vi "Load Layout.vi"(4 "PlotPane":refnum<vi>, 5 "MultiPlotPanel in":refnum<class "MultiPlotPanel.lvclass">, 6 "Subpanel Refs (ALL)":refnum<vi>[](array[refnum]), 7 "RocketPlotPanel Type":refnum<class "RocketPlotPanel.lvclass">, 8 "error in (no error)":errorcluster, 10 "file extension":string, 11 "Loop data in":T1 {"PanelMap"."Data"."Plot Bounds (%)"."Bottom (%)" format="%.2f"; "PanelMap"."Data"."Plot Bounds (%)"."Top (%)" format="%.2f"; "PanelMap"."Data"."Plot Bounds (%)"."Right (%)" format="%.2f"; "PanelMap"."Data"."Plot Bounds (%)"."Left (%)" format="%.2f"}) -> (0 "error out":errorcluster, 1 "Valid load?":bool, 2 "Filename":string, 3 "Loop data out":T1 {"PanelMap"."Data"."Plot Bounds (%)"."Bottom (%)" format="%.2f"; "PanelMap"."Data"."Plot Bounds (%)"."Top (%)" format="%.2f"; "PanelMap"."Data"."Plot Bounds (%)"."Right (%)" format="%.2f"; "PanelMap"."Data"."Plot Bounds (%)"."Left (%)" format="%.2f"})   [LabVIEW 2021, in "MultiStokePlot.lvlib" / "MultiPlotPanel.lvclass"]
uses:
  Classes/MultiPlotPanel/MultiPlotPanel.lvclass
  Loop Data.ctl
  <vilib>/IlluminatedG/IG OOPanel/OOPanel/Manager/Manager.lvclass
  Panel Map.ctl
  Panel Map Data.ctl
  <userlib>/bjustice/RocketPlot/Classes/RocketPlotPanel/RocketPlotPanel.lvclass
  Window Position.ctl
  <vilib>/IlluminatedG/IG OOPanel/OOPanel/Panel/Panel Events.ctl
  <vilib>/IlluminatedG/IG OOPanel/OOPanel/Panel/Visbility Event Data.ctl
  <vilib>/IlluminatedG/IG OOPanel/OOPanel/Visibility State.ctl
  <vilib>/IlluminatedG/IG OOPanel/OOPanel/Close Reason.ctl
  Classes/MultiPlotPanel/MultiPlotPanel.lvclass/MultiPlotPanel.ctl
  Window Position and plot number.ctl
  <userlib>/bjustice/RocketPlot/Classes/RocketPlotPanel/RocketPlotPanel.lvclass/RocketPlotPanel.ctl
  <userlib>/bjustice/RocketPlot/Classes/RocketPlotPanel/Read RocketPlotHandle.vi
  <userlib>/bjustice/RocketPlot/Classes/RocketPlotHandle/RocketPlotHandle.lvclass
  <vilib>/IlluminatedG/IG OOPanel/OOPanel/OOPanel.lvlib
  <vilib>/IlluminatedG/IG OOPanel/OOPanel/Panel/Panel.lvclass
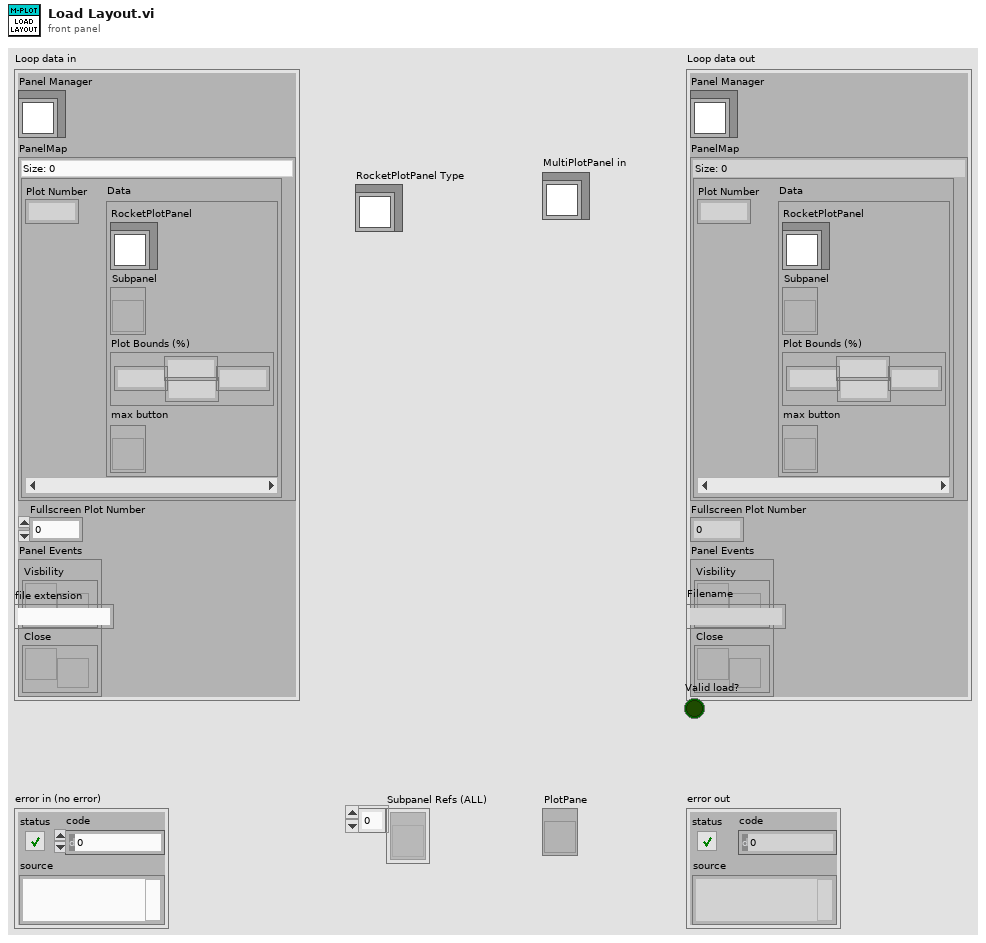
[diagram p1: front panel]
types:
  T1 = typedef "MultiStokePlot.lvlib/MultiPlotPanel.lvclass/Loop Data.ctl" = cluster{"Panel Manager":refnum<class "Manager.lvclass">, "PanelMap":T2, "Fullscreen Plot Number":i32, "Panel Events":T5}
  T2 = typedef "MultiStokePlot.lvlib/MultiPlotPanel.lvclass/Panel Map.ctl" = map{i32, T3}
  T3 = typedef "MultiStokePlot.lvlib/MultiPlotPanel.lvclass/Panel Map Data.ctl" = cluster{"RocketPlotPanel":refnum<class "RocketPlotPanel.lvclass">, "Subpanel":refnum<vi>, "Plot Bounds (%)":T4, "max button":refnum<vi>}
  T4 = typedef "MultiStokePlot.lvlib/MultiPlotPanel.lvclass/Window Position.ctl" = cluster{"Left (%)":dbl, "Top (%)":dbl, "Right (%)":dbl, "Bottom (%)":dbl}
  T5 = typedef "OOPanel.lvlib/Panel.lvclass/Panel Events.ctl" = cluster{"Visbility":refnum<user-event>, "Close":refnum<user-event>}
  T6 = typedef "MultiStokePlot.lvlib/MultiPlotPanel.lvclass/Window Position and plot number.ctl" = cluster{"Plot Number":i32, "Plot Bounds (%)":T4}
  T7 = typedef "MultiStokePlot.lvlib/MultiPlotPanel.lvclass/SinglePlotConfig.ctl" = cluster{"Plot Number":i32, "Plot Bounds (%)":T4, "RocketPlotConfig":T8}
  T8 = typedef "RocketPlot.lvlib/plot load data V2.ctl" = cluster{"plots":T9[], "X-axis":T11, "Y-axes":T11[], "General":T12}
  T9 = typedef "RocketPlot.lvlib/plot properties V2.ctl" = cluster{"attributes":T10, "Numeric":dbl, "Flatline?":bool}
  T10 = typedef "RocketPlot.lvlib/plot attributes V2.ctl" = cluster{"Plot Color":u32, "Point Style":u8, "Line Style":u8, "Plot Interpolation":u8, "Line Width":u8, "Bar Plot Style":u8, "Fill To":i16, "X Scale Index":u32, "Y Scale Index":u32, "Anti-aliased":bool, "Label Format":u8, "Digital Transition Type":u8, "Digital Transition Location":u8, "Digital Line Style":u8, "Fill/Point Color":u32, "Plot Name":string, "Visible":bool}
  T11 = typedef "RocketPlot.lvlib/Plot scale axis properties.ctl" = cluster{"Name Label.Text":string, "Style":u8, "Tick Colors:Minor Tick Color":u32, "Tick Colors:Tick Color":u32, "Marker Colors:Text Color":u32, "Grid Colors:Major Color":u32, "Grid Colors:Minor Color":u32, "Mapping Mode":u8, "Flipped":bool, "Name Label.Visible":bool, "Name Label.Text Colors:Text Color":u32, "Scale Fit":u8, "Range:Maximum":dbl, "Range:Minimum":dbl, "Offset and Multiplier:Multiplier":dbl, "Offset and Multiplier:Offset":dbl, "Name Label.Font:Size":u32, "Marker.Font:Size":u32, "Uniform Marker Spacing?":bool, "Format String":string}
  T12 = typedef "RocketPlot.lvlib/Plot general properties.ctl" = cluster{"Title":string, "Time to Plot":dbl, "Title.Visible":bool, "Sidebar.Visible":bool, "Plot Area:Colors:BG Color":u32, "X Scale.Plot Name":string, "X Scale.Use Plot Name":bool}
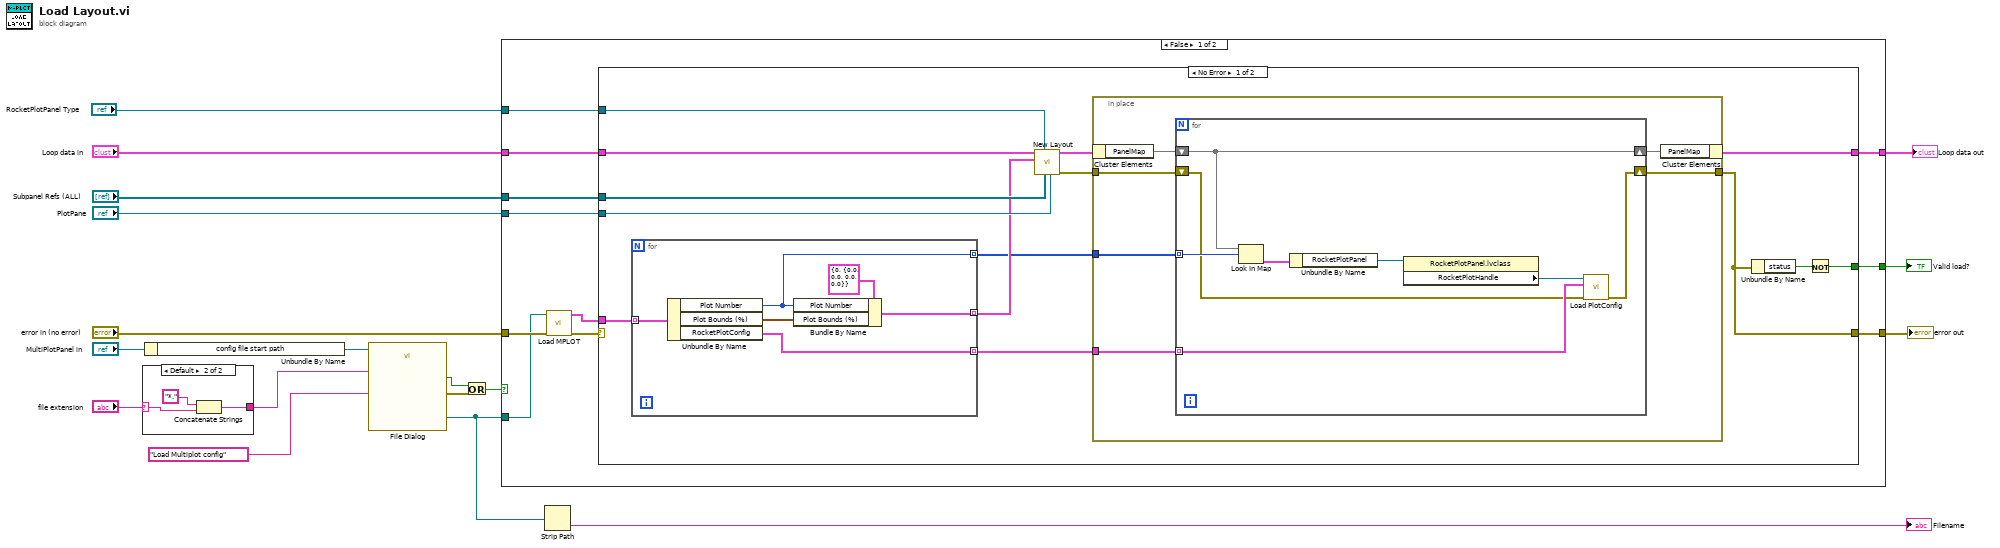
[diagram p0: block diagram]
diagram:
  n1 = case shown="Default" "file extension" {
    selector: "file extension" -> [w19 w21]
    tunnel: [w19 w20] -> w15
    frame "" {
    }
    frame Default {
      n2 = Concatenate Strings("*." ("string"), w21) -> (w20:string)
    }
  }
  n3 = Unbundle By Name("MultiPlotPanel in") -> ("config file start path"=w2:path)
  n4 = call "File Dialog"("start path"=w2, "prompt"="Load Multiplot config", "pattern (all files)"=w15) -> ("selected path"=w6:path, "cancelled"=w13:bool, "error out"=w12:errorcluster)  [unwired: 9 in, 1 out]
  n5 = Or(x=w13, y=w12) -> (x .or. y?=w11:bool)
  n6 = case shown="False" w11 {
    tunnel: w6 -> [w24 _]
    tunnel: [w29 w71] -> w16
    tunnel: "error in (no error)" -> [w28 w71]
    tunnel: "Loop data in" -> [w32 w70]
    tunnel: "Subpanel Refs (ALL)" -> [w31 _]
    tunnel: "PlotPane" -> [w30 _]
    tunnel: [w27 w70] -> w7
    tunnel: [w26 _] -> w4
    tunnel: "RocketPlotPanel Type" -> [w25 _]
    frame False {
      n7 = call "Load MPLOT.vi"("error in (no error)"=w28, "Filepath"=w24) -> ("error out"=w33:errorcluster, "RocketPlots"=w23:T7[])  [unwired: 8 in]
      n8 = case shown="No Error" w33 {
        selector: w33 -> [_ w69]
        tunnel: w23 -> [w44 _]
        tunnel: w32 -> [w47 w68]
        tunnel: w31 -> [w46 _]
        tunnel: w30 -> [w45 _]
        tunnel: [w37 w69] -> w29
        tunnel: [w38 w68] -> w27
        tunnel: [w35 _] -> w26
        tunnel: w25 -> [w34 _]
        frame No Error {
          n9 = for {
            tunnel: w44 -> [w53] mode=indexing
            tunnel: [w50] -> w43 mode=indexing
            tunnel: [w48] -> w40 mode=indexing
            tunnel: [w49] -> w41 mode=indexing
            n10 = Unbundle By Name(w53) -> ("Plot Number"=w49:i32, "Plot Bounds (%)"=w51:T4, "RocketPlotConfig"=w48:T8)
            n11 = Bundle By Name(cluster=T6 {"Plot Number"=0, "Plot Bounds (%)"={"Left (%)"=0.0, "Top (%)"=0.0, "Right (%)"=0.0, "Bottom (%)"=0.0}} ("Cluster"), "Plot Number"=w49, "Plot Bounds (%)"=w51) -> (w50:T6)
          }
          n12 = call "New Layout.vi"("PlotPane"=w45, "Subpanel Refs (ALL)"=w46, "RocketPlotPanel Type"=w34, "Layout"=w43, "Loop data in"=w47) -> ("error out"=w39:errorcluster, "Loop data out"=w42:T1)  [unwired: 5 in]
          n13 = in-place {
            in-place-border: w41 -> [w57]
            in-place-border: w40 -> [w56]
            in-place-border: w39 -> [w55]
            in-place-border: [w54] -> w37
            n14 = in-place-cluster #1(w42) -> ("PanelMap"=w59:T2)
            n15 = for {
              shift-right: [w62] -> w58
              shift-left: w59 -> [w62]
              tunnel: w57 -> [w64] mode=indexing
              tunnel: w56 -> [w67] mode=indexing
              shift-right: [w60] -> w54
              shift-left: w55 -> [w61]
              n16 = Look In Map(map=w62, key=w64) -> (value=w63:T3)  [unwired: 1 in, 1 out]
              n17 = Unbundle By Name(w63) -> ("RocketPlotPanel"=w66:refnum<class "RocketPlotPanel.lvclass">)
              n18 = property class="RocketPlotPanel.lvclass"(reference=w66) -> ("RocketPlotHandle"=w65:refnum<class "RocketPlotHandle.lvclass">)  [unwired: 1 in, 2 out]
              n19 = call <userlib>:"Load PlotConfig.vi"("error in (no error)"=w61, "Plot config"=w67, "BluePlotHandle in"=w65) -> ("error out"=w60:errorcluster)  [unwired: 7 in, 1 out]
            }
            n20 = in-place-cluster #1("PanelMap"=w58) -> (w38:T1)
          }
          n21 = Unbundle By Name(w37) -> ("status"=w36:bool)
          n22 = Not(x=w36) -> (.not. x?=w35:bool)
        }
        frame Error {
        }
      }
    }
    frame True {
    }
  }
  "Loop data out" <- w7
  "error out" <- w16
  "Valid load?" <- w4
  n23 = Strip Path(path=w6) -> (name=→"Filename":string)  [unwired: 1 out]
